vi "SendToMod.vi"(8 "error in (no error)":errorcluster, 9 "Data":variant, 10 "Command":T1, 11 "JQMHStartup in":refnum<class "RQMHStartup.lvclass">) -> (0 "error out":errorcluster, 3 "JQMHStartup out":refnum<class "RQMHStartup.lvclass">)   [LabVIEW 2024, in "RQMHStartup.lvclass"]
uses:
  RQMHStartup.lvclass
  Command.ctl
  Message.ctl
  RQMHStartup.lvclass/RQMHStartup.ctl
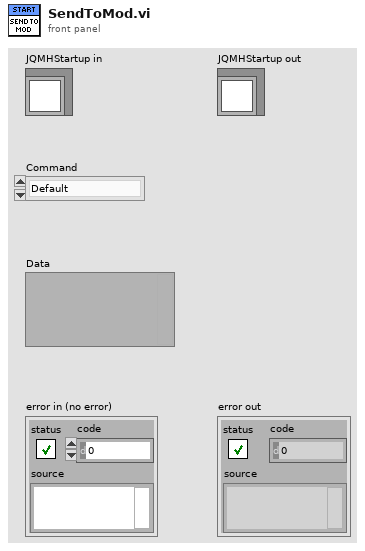
[diagram p1: front panel]
types:
  T1 = typedef "RQMHStartup.lvclass/Command.ctl" = enum16{"Default", "No Override", "Error", "ACK Created", "ACK Mod Reg", "ACK Caller Reg"}
  T2 = typedef "RQMHStartup.lvclass/Message.ctl" = cluster{"Command":T1, "Data":variant}
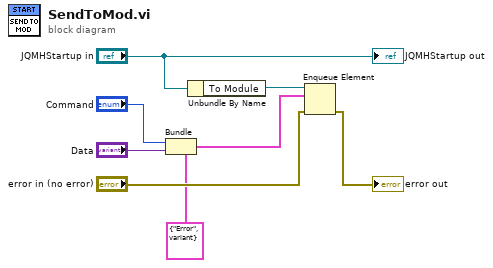
[diagram p0: block diagram]
diagram:
  n1 = Bundle(cluster=T2 {"Command"=enum."Error", "Data"=variant} ("element"), "Command"="Command", "Data"="Data") -> (w3:T2)
  n2 = Unbundle By Name("JQMHStartup in") -> ("To Module"=w5:refnum<queue>)
  n3 = Enqueue Element(queue=w5, element=w3, error in (no error)="error in (no error)") -> (error out=→"error out":errorcluster)  [unwired: 1 in, 2 out]
  "JQMHStartup out" <- "JQMHStartup in"
